vi "savingPrepDataForDisp_bin_01.vi"(8 "error in (no error)":errorcluster, 9 "buffer in":i16[](array[numeric]), 10 "Channels to read":i32) -> (0 "error out":errorcluster, 2 "Array":dbl[][](array[numeric]))   [LabVIEW 2021]
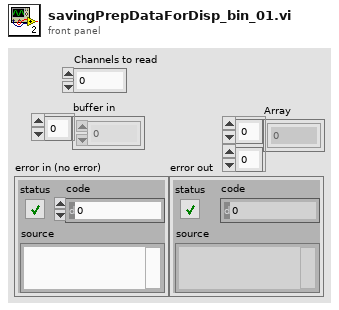
[diagram p1: front panel]
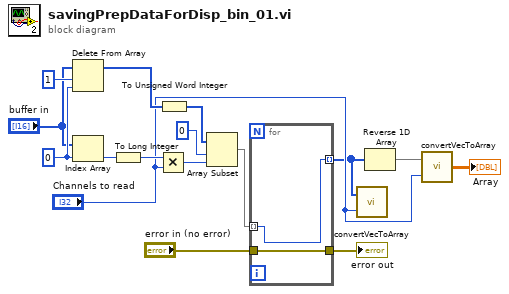
[diagram p0: block diagram]
diagram:
  w15 = 0 ("index")
  n1 = Delete From Array(array="buffer in", length=1, index=w15) -> (array with subset deleted=w16:i16[])  [unwired: 1 out]
  n2 = Index Array(array="buffer in", index=w15) -> (element=w7:i16)
  n3 = To Long Integer(number=w7) -> (32bit integer=w8:i32)
  n4 = Multiply(x=w8, y="Channels to read") -> (x*y=w9:i32)
  n5 = To Unsigned Word Integer(number=w16) -> (unsigned 16bit integer=w10:u16[])
  n6 = Array Subset(array=w10, index=0, length=w9) -> (w2:u16[])
  n7 = for {
    tunnel: w2 -> [w17] mode=indexing
    tunnel: [w17] -> w3 mode=indexing
    tunnel: "error in (no error)" -> [w18]
    tunnel: [w18] -> w1
  }
  "error out" <- w1
  n8 = call "convertVecToArray.vi"("Channels"="Channels to read", "buffer in"=w3) -> ()  [unwired: 1 out]
  n9 = Reverse 1D Array(array=w3) -> (reversed array=w6:u16[])
  n10 = call "convertVecToArray.vi"("Channels"="Channels to read", "buffer in"=w6) -> ("Array"=→"Array":dbl[][])
